vi "MouseInput.vi"() -> ()   [LabVIEW 2018]
uses:
  <vilib>/Utility/inputDevices.llb/mouseAcquire.vi
panel:
  out "Mouse Position\nCluster":T1
  out "Mouse Button Cluster":cluster{"Left Button":bool, "Right Button":bool}
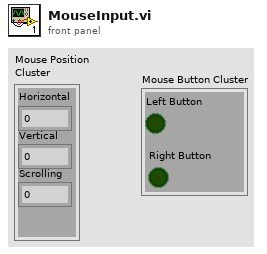
[diagram p1: front panel]
types:
  T1 = cluster{"Horizontal":i32, "Vertical":i32, "Scrolling":i32}
  T2 = cluster{"button 1":bool, "button 2":bool, "button 3":bool, "button 4":bool}
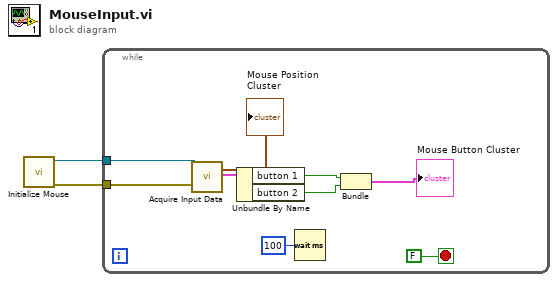
[diagram p0: block diagram]
diagram:
  n1 = call <vilib>:"Initialize Mouse.vi"() -> ("error out"=w1:errorcluster, "device ID"=w2:refnum<k1>)  [unwired: 10 in]
  n2 = while {
    tunnel: w2 -> [w10]
    tunnel: w1 -> [w9]
    stop <- FALSE stop-if-true
    n3 = call-poly <vilib>:"Acquire Input Data.vi"("device ID"=w10, "error in (no error)"=w9) -> ("axis info"=→"Mouse Position\nCluster":T1, "button info"=w8:T2)  [unwired: 14 in, 2 out]
    n4 = Unbundle By Name(w8) -> ("button 1"=w7:bool, "button 2"=w6:bool)
    n5 = Wait (ms)(milliseconds to wait=u32 100) -> ()  [unwired: 1 out]
    n6 = Bundle("button 1"=w7, "button 2"=w6) -> (→"Mouse Button Cluster":cluster{"button 1":bool, "button 2":bool})  [unwired: 1 in]
  }
